vi "BIO_do_connect_accept.vi"(7 "Timeout (10000ms)":u32=10000, 8 "error in (no error)":errorcluster, 11 "BIO in":refnum<class "BIO.lvclass">) -> (0 "error out":errorcluster, 3 "BIO out":refnum<class "BIO.lvclass">)   [LabVIEW 2013, in "SSL_Lib.lvlib" / "BIO.lvclass"]
uses:
  BIO.lvclass
  SSL-Lib/SSL-Lib.lvclass
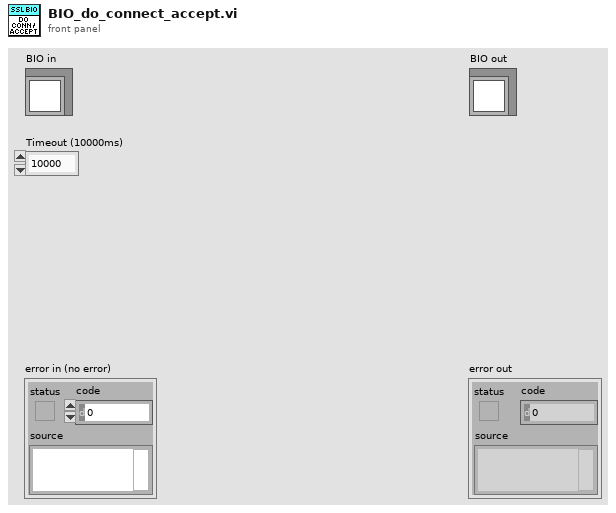
[diagram p1: front panel]
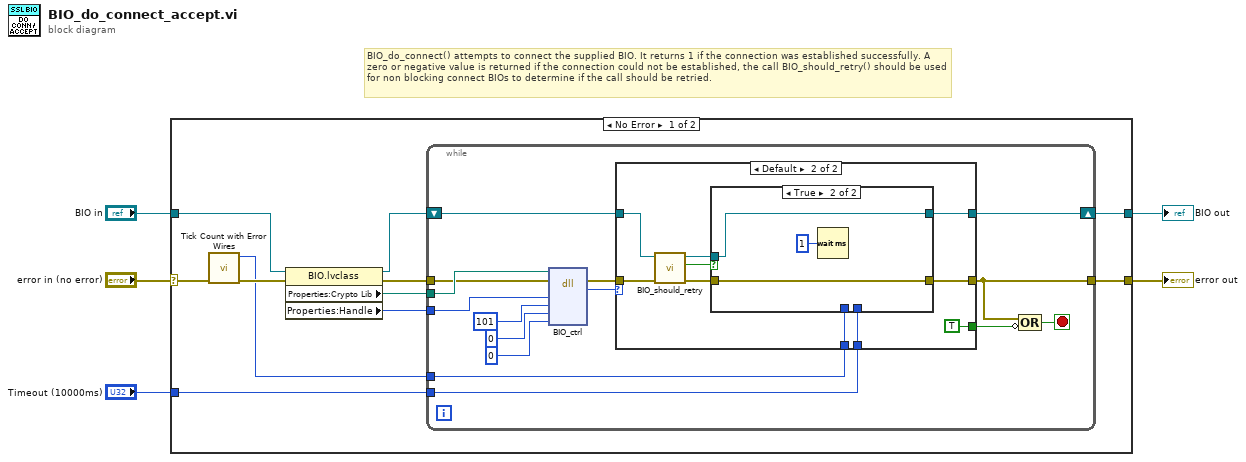
[diagram p0: block diagram]
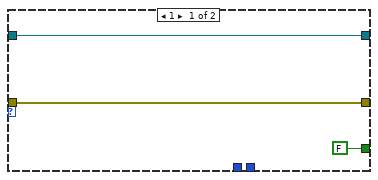
[diagram p2: hidden frame]
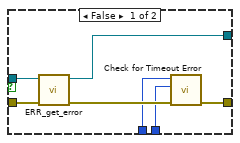
[diagram p3: hidden frame]
diagram:
  # "BIO_do_connect() attempts to connect the supplied BIO. It returns 1 if the connection was established successfully. A zero or negative value is returned if the connection could not be established, the call BIO_should_retry() should be used for non blocking connect BIOs to determine if the call should be retried."
  n1 = case shown="No Error" "error in (no error)" {
    selector: "error in (no error)" -> [w10 w56]
    tunnel: [w13 w56] -> w4
    tunnel: [w11 w55] -> w2
    tunnel: "BIO in" -> [w9 w55]
    tunnel: "Timeout (10000ms)" -> [w6 _]
    frame No Error {
      n2 = call "Tick Count with Error Wires.vi"("error in (no error)"=w10) -> ("error out"=w8:errorcluster, "millisecond timer value"=w7:u32)  [unwired: 9 in]
      n3 = property class="BIO.lvclass"(reference=w9, error in=w8) -> (reference out=w12:refnum<class "BIO.lvclass">, error out=w14:errorcluster, "Properties:Crypto Lib"=w15:path, "Properties:Handle"=w16:u64)
      n4 = while {
        tunnel: w16 -> [w28]
        tunnel: w15 -> [w27]
        shift-right: [w23] -> w11
        shift-left: w12 -> [w24]
        tunnel: w7 -> [w18]
        tunnel: w6 -> [w19]
        tunnel: w14 -> [w26]
        tunnel: [w17] -> w13
        stop <- w21 stop-if-true
        n5 = dll-call lib="C:/Program Files (x86)/National Instruments/Shared/nissl/NIlibeay32.dll" fn="BIO_ctrl"(path in=w27, error in=w26, "BIO"=w28, "cmd"=101, "larg"=0, "parg"=0 ("larg")) -> (error out=w25:errorcluster, "return type"=w22:i32)  [unwired: 5 in, 1 out]
        n6 = case shown="Default" w22 {
          tunnel: w25 -> [w34 w44]
          tunnel: w24 -> [w33 w43]
          tunnel: [w33 w40] -> w23
          tunnel: [w34 w37] -> w17
          tunnel: [FALSE ("Should retry") TRUE ("Should retry")] -> w20
          tunnel: w19 -> [_ w39]
          tunnel: w18 -> [_ w38]
          frame 1 {
          }
          frame Default {
            n7 = call "BIO_should_retry.vi"("error in (no error)"=w44, "BIO in"=w43) -> ("error out"=w42:errorcluster, "Should retry"=w35:bool, "BIO out"=w41:refnum<class "BIO.lvclass">)  [unwired: 7 in]
            n8 = case shown="True" w35 {
              tunnel: w42 -> [w51 w53]
              tunnel: w41 -> [w50 w54]
              tunnel: [w49 w54] -> w40
              tunnel: w39 -> [w47 _]
              tunnel: w38 -> [w46 _]
              tunnel: [w45 w53] -> w37
              frame False {
                n9 = call "ERR_get_error.vi"("error in (no error)"=w51, "SSL-Lib in"=w50) -> ("error out"=w48:errorcluster, "SSL-Lib out"=w49:refnum<class "BIO.lvclass">)  [unwired: 8 in]
                n10 = call "Check for Timeout Error.vi"("error in (no error)"=w48, "Timeout (10000ms)"=w47, "t0"=w46) -> ("error out"=w45:errorcluster)  [unwired: 8 in]
              }
              frame True {
                n11 = Wait (ms)(milliseconds to wait=u32 1) -> ()  [unwired: 1 out]
              }
            }
          }
        }
        n12 = Compound Arithmetic op=OR(w17, invert w20) -> (w21:bool)
      }
    }
    frame Error {
    }
  }
  "error out" <- w4
  "BIO out" <- w2
